vi "Configure OSC CStandard query.vi"(8 "error in (no error)":errorcluster, 9 "Step":u16=1 min=1 max=99 step=1, 11 "VISA resource in":refnum<visa-resource-name>) -> (0 "error out":errorcluster, 1 "Cs":string, 3 "VISA resource out":refnum<visa-resource-name>)   [LabVIEW 2025]
doc: "This VI set the OPEN limit for Open/Short Circuit (OSC) test mode.\nRange: 0.1 to 1, step 0.1"
uses:
  <instrlib>/Chroma 19052/Chroma 19052.lvlib
panel:
  # "[F]"
  # "Query OSC CST value"
  # "Range 1:  0.001nF - 9.999nF\nRange 2:  0.01nF - 99.99nF\nRange 3:  0.1nF - 500.0nF"
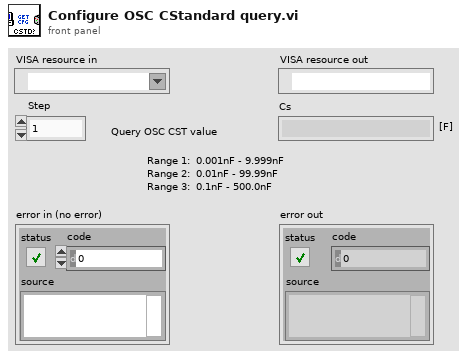
[diagram p1: front panel]
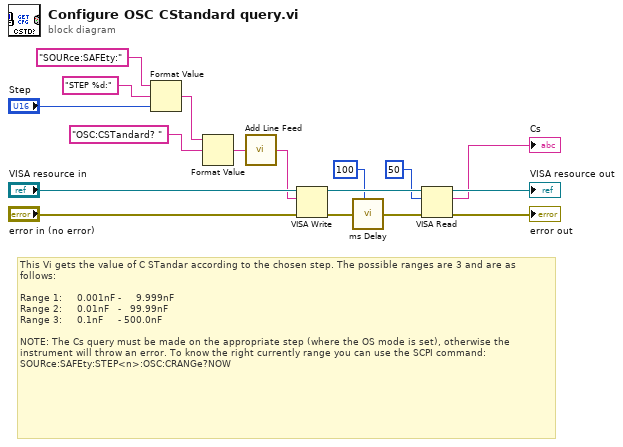
[diagram p0: block diagram]
diagram:
  # "This Vi gets the value of C STandar according to the chosen step. The possible ranges are 3 and are as follows:\n\nRange 1:     0.001nF -     9.999nF\nRange 2:     0.01nF   -   99.99nF\nRange 3:     0.1nF     - 500.0nF\n\nNOTE: The Cs query must be made on the appropriate step (where the OS mode is set), otherwise the \ninstrument will throw an error. To know the right currently range you can use the SCPI command:\nSOURce:SAFEty:STEP<n>:OSC:CRANGe?NOW"
  n1 = Format Value(string ("")="SOURce:SAFEty:", format string="STEP %d:", value (0)="Step") -> (output string=w8:string)
  n2 = Format Value(string ("")=w8, format string="OSC:CSTandard? ") -> (output string=w5:string)  [unwired: 1 in]
  n3 = call <instrlib>:"Add Line Feed.vi"("Command string"=w5) -> ("Concatenated string"=w1:string)  [unwired: 4 in]
  n4 = VISA Write(VISA resource name="VISA resource in", write buffer=w1, error in (no error)="error in (no error)") -> (VISA resource name out=w7:refnum<visa-resource-name>, error out=w4:errorcluster)  [unwired: 1 out]
  n5 = call <instrlib>:"ms Delay.vi"("miliseconds to wait"=u32 100, "error in (no error)"=w4) -> ("error out"=w3:errorcluster)  [unwired: 6 in, 1 out]
  n6 = VISA Read(VISA resource name=w7, byte count=u32 50, error in (no error)=w3) -> (VISA resource name out=→"VISA resource out":refnum<visa-resource-name>, read buffer=→"Cs":string, error out=→"error out":errorcluster)  [unwired: 1 out]
